vi "Climber.vi"   [LabVIEW 2020]
uses:
  <vilib>/Rock Robotics/WPI/Solenoid/WPI_SolenoidValue.ctl
  <vilib>/Rock Robotics/WPI/Utilities/WPI_GetSetVariantRefNum.vi
  <vilib>/Rock Robotics/WPI/Solenoid/WPI_SolenoidSetEnum.vi
types:
  T1 = typedef "WPI_JoystickDevRef.ctl" = cluster{"Device":T2}
  T2 = typedef "WPI_JoystickDeviceEnum.ctl" = enum16{"USB 0", "USB 1", "USB 2", "USB 3", "USB 4", "USB 5"}
  T3 = typedef "WPI_SolenoidValue.ctl" = enum16{"Off", "On", "Forward", "Reverse"}
  T4 = typedef "WPI_SolenoidDevRef.ctl" = cluster{"DevStatus":errorcluster, "Pneumatics Control Module":u8, "Forward Solenoid Channel":T5, "Reverse Solenoid Channel":T5}
  T5 = typedef "WPI_SolenoidChannel.ctl" = enum8{"Solenoid 0", "Solenoid 1", "Solenoid 2", "Solenoid 3", "Solenoid 4", "Solenoid 5", "Solenoid 6", "Solenoid 7", "Solenoid 8", "Solenoid 9", "Solenoid 10", "Solenoid 11", "Solenoid 12", "Solenoid 13", "Solenoid 14", "Solenoid 15", "Invalid"}
  T6 = typedef "WPI_MotorControlDeviceRef.ctl" = cluster{"DeviceStatus":errorcluster, "Type":T7, "PWM":cluster{"PWM Channel":T8, "DeadBand":T9}, "CAN":cluster{"Device Number":u8, "SetOutput VI Ref":variant, "GetOutput VI Ref":variant, "Enable VI Ref":variant, "Disable VI Ref":variant, "Data":variant}, "Invert":bool, "DIO PWM":cluster{"PWM \"Enable\" Channel":T8, "DIOChannel":T10, "PWM Rate":dbl}}
  T7 = typedef "WPI_MotorControlType.ctl" = enum16{"PWM", "CAN", "DIO PWM"}
  T8 = typedef "FPGA_DIOPWMChannel.ctl" = enum8{"PWM 0", "PWM 1", "PWM 2", "PWM 3", "PWM 4", "PWM 5", "PWM 6", "PWM 7", "PWM 8", "PWM 9", "PWM MXP 0", "PWM MXP 1", "PWM MXP 2", "PWM MXP 3", "PWM MXP 4", "PWM MXP 5", "PWM MXP 6", "PWM MXP 7", "PWM MXP 8", "PWM MXP 9", "Invalid"}
  T9 = typedef "WPI_PWMDeadband.ctl" = cluster{"Name":string, "maxPositivePwm":i32, "minPositivePwm":i32, "centerPwm":i32, "maxNegativePwm":i32, "minNegativePwm":i32, "angularRange":u16}
  T10 = typedef "FPGA_DIOChannel.ctl" = enum8{"DIO 0", "DIO 1", "DIO 2", "DIO 3", "DIO 4", "DIO 5", "DIO 6", "DIO 7", "DIO 8", "DIO 9", "DIO MXP 0", "DIO MXP 1", "DIO MXP 2", "DIO MXP 3", "DIO MXP 4", "DIO MXP 5", "DIO MXP 6", "DIO MXP 7", "DIO MXP 8", "DIO MXP 9", "DIO MXP 10", "DIO MXP 11", "DIO MXP 12", "DIO MXP 13", "DIO MXP 14", "DIO MXP 15", "SPI Port CS1", "SPI Port CS2", "SPI Port CS3", "SPI Port MISO", "SPI Port MOSI", "Invalid"}
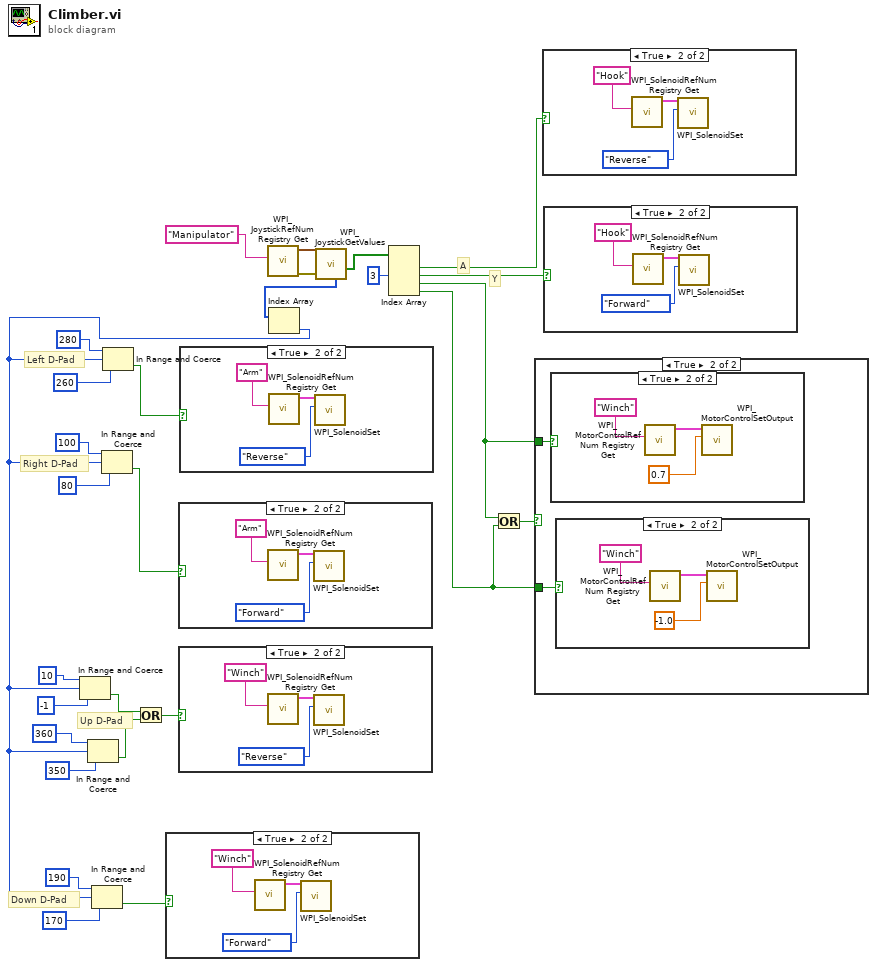
[diagram p0: block diagram]
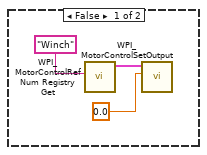
[diagram p2: hidden frame]
diagram:
  # "Down D-Pad"
  # "Up D-Pad"
  # "Right D-Pad"
  # "Left D-Pad"
  # "Y"
  # "A"
  n1 = call <vilib>:"WPI_JoystickRefNum Registry Get.vi"("refnum name"="Manipulator") -> ("error out"=w27:errorcluster, "JoystickDevRef"=w28:T1)  [unwired: 1 in, 8 out]
  n2 = call <vilib>:"WPI_JoystickGetValues.vi"("error in (no error)"=w27, "JoystickDevRef"=w28) -> ("Buttons"=w25:bool[], "POVs"=w26:i16[])  [unwired: 5 in, 3 out]
  n3 = Index Array(array=w26) -> (element=w9:i16)  [unwired: 1 in]
  n4 = In Range and Coerce(upper limit=i16 10, x=w9, lower limit=i16 -1) -> (In Range?=w8:bool)  [unwired: 1 out]
  n5 = In Range and Coerce(upper limit=i16 360, x=w9, lower limit=i16 350) -> (In Range?=w7:bool)  [unwired: 1 out]
  n6 = In Range and Coerce(upper limit=i16 190, x=w9, lower limit=i16 170) -> (In Range?=w5:bool)  [unwired: 1 out]
  n7 = In Range and Coerce(upper limit=i16 100, x=w9, lower limit=i16 80) -> (In Range?=w16:bool)  [unwired: 1 out]
  n8 = In Range and Coerce(upper limit=i16 280, x=w9, lower limit=i16 260) -> (In Range?=w19:bool)  [unwired: 1 out]
  n9 = Or(x=w8, y=w7) -> (x .or. y?=w6:bool)
  n10 = case shown="True" w5 {
    frame False {
    }
    frame True {
      n11 = call <vilib>:"WPI_SolenoidRefNum Registry Get.vi"("refnum name"="Winch") -> ("SolenoidDevRef"=w31:T4)  [unwired: 9 in, 1 out]
      n12 = call-poly <vilib>:"WPI_SolenoidSet.vi"("Value"=WPI_SolenoidValue."Forward", "SolenoidDevRef"=w31) -> ()  [unwired: 8 in, 2 out]
    }
  }
  n13 = case shown="True" w16 {
    frame False {
    }
    frame True {
      n14 = call <vilib>:"WPI_SolenoidRefNum Registry Get.vi"("refnum name"="Arm") -> ("SolenoidDevRef"=w34:T4)  [unwired: 9 in, 1 out]
      n15 = call-poly <vilib>:"WPI_SolenoidSet.vi"("Value"=WPI_SolenoidValue."Forward", "SolenoidDevRef"=w34) -> ()  [unwired: 8 in, 2 out]
    }
  }
  n16 = case shown="True" w6 {
    frame False {
    }
    frame True {
      n17 = call <vilib>:"WPI_SolenoidRefNum Registry Get.vi"("refnum name"="Winch") -> ("SolenoidDevRef"=w37:T4)  [unwired: 9 in, 1 out]
      n18 = call-poly <vilib>:"WPI_SolenoidSet.vi"("Value"=WPI_SolenoidValue."Reverse", "SolenoidDevRef"=w37) -> ()  [unwired: 8 in, 2 out]
    }
  }
  n19 = case shown="True" w19 {
    frame False {
    }
    frame True {
      n20 = call <vilib>:"WPI_SolenoidRefNum Registry Get.vi"("refnum name"="Arm") -> ("SolenoidDevRef"=w40:T4)  [unwired: 9 in, 1 out]
      n21 = call-poly <vilib>:"WPI_SolenoidSet.vi"("Value"=WPI_SolenoidValue."Reverse", "SolenoidDevRef"=w40) -> ()  [unwired: 8 in, 2 out]
    }
  }
  n22 = Index Array(array=w25, index #2=3 ("index")) -> (element #1=w22:bool, element #2=w23:bool, element #3=w3:bool, element #4=w2:bool)  [unwired: 3 in]
  n23 = Or(x=w3, y=w2) -> (x .or. y?=w4:bool)
  n24 = case shown="True" w4 {
    tunnel: w3 -> [_ w45]
    tunnel: w2 -> [_ w44]
    frame False {
      n25 = call <vilib>:"WPI_MotorControlRefNum Registry Get.vi"("refnum name"="Winch") -> ("MotorControlDevRef"=w43:T6)  [unwired: 9 in, 1 out]
      n26 = call <vilib>:"WPI_MotorControlSetOutput.vi"("Output"=0.0, "MotorControlDevRef"=w43) -> ()  [unwired: 7 in, 3 out]
    }
    frame True {
      n27 = case shown="True" w45 {
        frame False {
        }
        frame True {
          n28 = call <vilib>:"WPI_MotorControlRefNum Registry Get.vi"("refnum name"="Winch") -> ("MotorControlDevRef"=w51:T6)  [unwired: 9 in, 1 out]
          n29 = call <vilib>:"WPI_MotorControlSetOutput.vi"("Output"=0.7, "MotorControlDevRef"=w51) -> ()  [unwired: 7 in, 3 out]
        }
      }
      n30 = case shown="True" w44 {
        frame False {
        }
        frame True {
          n31 = call <vilib>:"WPI_MotorControlRefNum Registry Get.vi"("refnum name"="Winch") -> ("MotorControlDevRef"=w48:T6)  [unwired: 9 in, 1 out]
          n32 = call <vilib>:"WPI_MotorControlSetOutput.vi"("Output"=-1.0, "MotorControlDevRef"=w48) -> ()  [unwired: 7 in, 3 out]
        }
      }
    }
  }
  n33 = case shown="True" w22 {
    frame False {
    }
    frame True {
      n34 = call <vilib>:"WPI_SolenoidRefNum Registry Get.vi"("refnum name"="Hook") -> ("SolenoidDevRef"=w54:T4)  [unwired: 9 in, 1 out]
      n35 = call-poly <vilib>:"WPI_SolenoidSet.vi"("Value"=WPI_SolenoidValue."Reverse", "SolenoidDevRef"=w54) -> ()  [unwired: 8 in, 2 out]
    }
  }
  n36 = case shown="True" w23 {
    frame False {
    }
    frame True {
      n37 = call <vilib>:"WPI_SolenoidRefNum Registry Get.vi"("refnum name"="Hook") -> ("SolenoidDevRef"=w57:T4)  [unwired: 9 in, 1 out]
      n38 = call-poly <vilib>:"WPI_SolenoidSet.vi"("Value"=WPI_SolenoidValue."Forward", "SolenoidDevRef"=w57) -> ()  [unwired: 8 in, 2 out]
    }
  }
